vi "Add Instr Configuration.vi"(8 "error in (no error)":errorcluster, 10 "Instr Configuration":string, 11 "Configurator Actor:Configuration UI Actor in":refnum<class "Configuration UI Actor.lvclass">) -> (0 "error out":errorcluster, 3 "Configurator Actor:Configuration UI Actor out":refnum<class "Configuration UI Actor.lvclass">)   [LabVIEW 2023, in "Configuration UI Actor.lvlib" / "Configuration UI Actor.lvclass"]
uses:
  Configuration UI Actor.lvclass
  Configuration UI Actor.lvclass/Configuration UI Actor.ctl
  <vilib>/Utility/miscctls.llb/LVMapReplaceAction.ctl
  00509a2b-7146-4dc8-88e7-3ca79c2a51b2.vi
  <vilib>/JDP Science/JSONtext/Find Item.vi
  <vilib>/JDP Science/JSONtext/Next JSON Value.vi
  <vilib>/JDP Science/JSONtext/String Subset.vi
  <vilib>/JDP Science/JSONtext/Parsing/Advance past next JSON Value (inlined COPY).vi
  <vilib>/JDP Science/JSONtext/Parsing/Advance past whitespace.vi
  <vilib>/JDP Science/JSONtext/Parsing/Advance past String.vi
  <vilib>/JDP Science/JSONtext/Parsing/Advance past Number.vi
  <vilib>/JDP Science/JSONtext/Parsing/Advance past Line Ending.vi
  <vilib>/JDP Science/JSONtext/Parsing/Parse Full Path or Item Name.vi
  <vilib>/JDP Science/JSONtext/Parsing/Advance past Array.vi
  <vilib>/JDP Science/JSONtext/Parsing/Advance past Object.vi
  <vilib>/JDP Science/JSONtext/support/Error Cluster From Code.vi
  <vilib>/JDP Science/JSONtext/Offset/Find Item Locations by Path.vi
  <vilib>/JDP Science/JSONtext/JSON text to Variant.vi
  <vilib>/Utility/error.llb/Error Cluster From Error Code.vi
  <vilib>/JDP Science/JSONtext/LVClass Serializer/JSONtext LVClass Serializer.lvclass
  <vilib>/ErrorRing/Error Ring.xnode
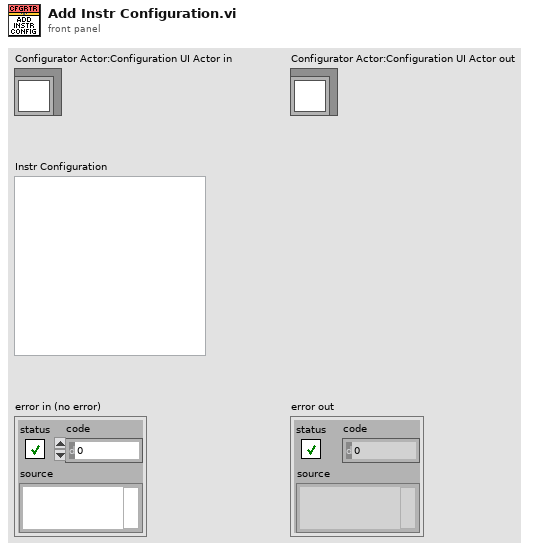
[diagram p1: front panel]
types:
  T1 = typedef "LVMapReplaceAction.ctl" = enum32{"Modify Entry only if found", "Add or Modify Entry", "Delete Entry"}
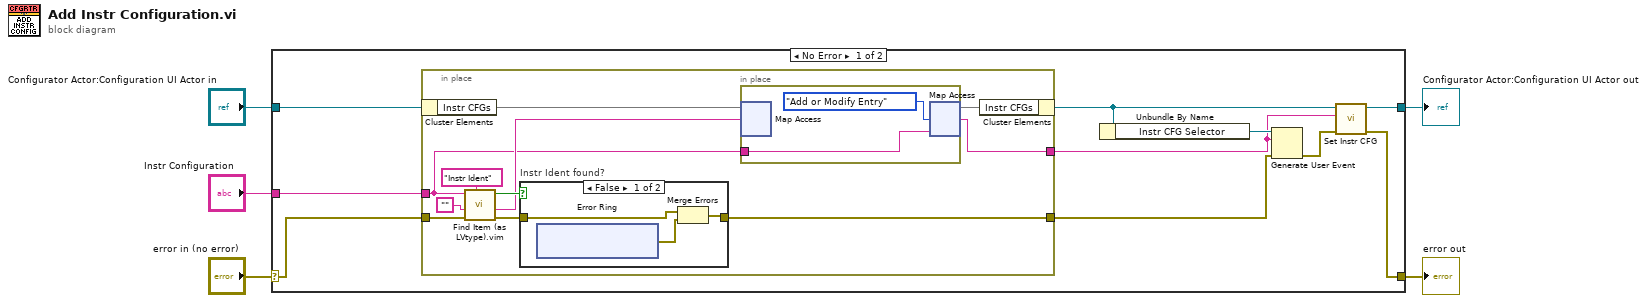
[diagram p0: block diagram]
diagram:
  n1 = case shown="No Error" "error in (no error)" {
    selector: "error in (no error)" -> [w12 w39]
    tunnel: [w7 w39] -> w4
    tunnel: [w8 w38] -> w2
    tunnel: "Configurator Actor:Configuration UI Actor in" -> [w15 w38]
    tunnel: "Instr Configuration" -> [w14 _]
    frame No Error {
      n2 = in-place {
        in-place-border: w14 -> [w19]
        in-place-border: w12 -> [w24]
        in-place-border: [w18] -> w11
        in-place-border: [w16] -> w6
        n3 = in-place-cluster #1(w15) -> ("Instr CFGs"=w26:map{string, string})
        n4 = call "Find Item (as LVtype).vim"("$Path or Item Name"="Instr Ident", "error in (no error)"=w24, "Data Type and Default Value"="", "JSON"=w19) -> ("error out"=w21:errorcluster, "Data"=w20:string, "Found"=w22:bool)  [unwired: 4 in, 1 out]
        n5 = case "Instr Ident found?" shown="False" w22 {
          tunnel: [w27 w35] -> w18
          tunnel: w21 -> [w28 w35]
          frame False {
            n6 = xnode "Error Ring"() -> ("error out"=w29:errorcluster)
            n7 = Merge Errors(w28, w29) -> (w27:errorcluster)
          }
          frame True {
          }
        }
        n8 = in-place {
          in-place-border: w19 -> [w36]
          n9 = in-place-map #2(w26, w20) -> ()  [unwired: 1 in, 2 out]
          n10 = in-place-map #2(w36, LVMapReplaceAction."Add or Modify Entry" ("action")) -> (w17:map{string, string}, w16:string)  [unwired: 1 out]
        }
        n11 = in-place-cluster #1("Instr CFGs"=w17) -> (w9:refnum<class "Configuration UI Actor.lvclass">)
      }
      n12 = Unbundle By Name(w9) -> ("Instr CFG Selector"=w13:refnum<user-event>)
      n13 = Generate User Event(user event=w13, event data cluster=w6, error in=w11) -> (error out=w10:errorcluster)  [unwired: 1 in, 1 out]
      n14 = call-dynamic "Set Instr CFG.vi"("Error In"=w10, "Instr Ident"=w6, "object in"=w9) -> ("Error Out"=w7:errorcluster, "object out"=w8:refnum<class "Configuration UI Actor.lvclass">)  [unwired: 7 in]
    }
    frame Error {
    }
  }
  "error out" <- w4
  "Configurator Actor:Configuration UI Actor out" <- w2
